vi "generate_random_rectangular_grid_and_word_list.vi"(7 "size (rows, columns)":i32[](array[numeric])=[300, 300], 9 "Min Word Length":u64=10, 10 "Max Word Length":u64=150, 11 "number of words":i32=300) -> (2 "Words":string[](array[string]), 3 "Grid":string[][](array[string]))   [LabVIEW 2020]
uses:
  <vilib>/numeric/Random Number (Range) U64.vi
  Letter Index--cluster.ctl
panel:
  # "From: Christian Altenbach\n https://forums.ni.com/t5/LabVIEW-Champions-Directory/LabVIEW-Champion-Christian-Altenbach/ta-p/3495223"
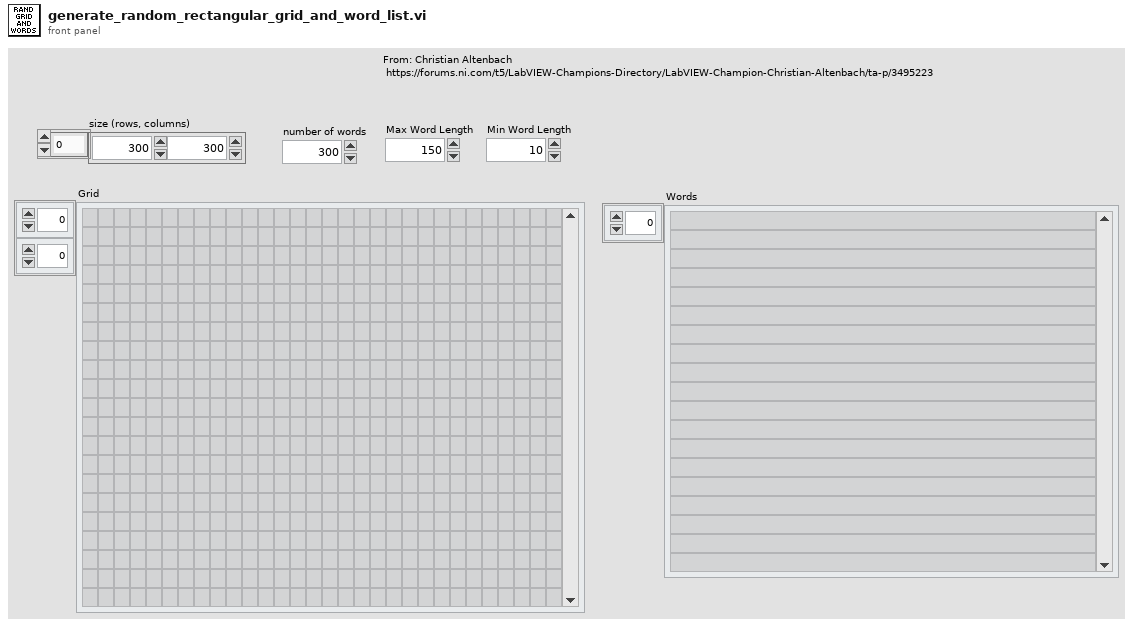
[diagram p1: front panel]
types:
  T1 = typedef "Letter Index--cluster.ctl" = cluster{"Row":i32, "Column":i32}
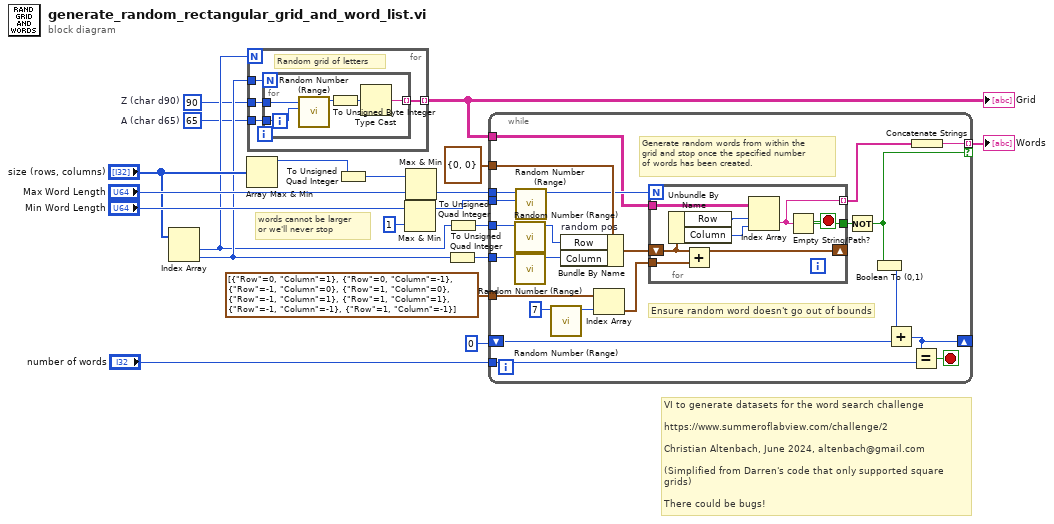
[diagram p0: block diagram]
diagram:
  w1 = u64 65  # A (char d65)
  w2 = u64 90  # Z (char d90)
  # "VI to generate datasets for the word search challenge\n\nhttps://www.summeroflabview.com/challenge/2\n\nChristian Altenbach, June 2024, altenbach@gmail.com\n\n(Simplified from Darren's code that only supported square grids)\n\nThere could be bugs!"
  # "words cannot be larger\nor we'll never stop"
  n1 = Index Array(array="size (rows, columns)") -> (element #1=w8:i32, element #2=w9:i32)  [unwired: 2 in]
  n2 = Array Max & Min(array="size (rows, columns)") -> (max value=w5:i32)  [unwired: 3 out]
  n3 = for {
    N: w8 -> [_]
    tunnel: [w24] -> w20 mode=indexing
    tunnel: w9 -> [w23]
    tunnel: w2 -> [w22]
    tunnel: w1 -> [w21]
    # "Random grid of letters"
    n4 = for {
      N: w23 -> [_]
      tunnel: [w27] -> w24 mode=indexing
      tunnel: w22 -> [w26]
      tunnel: w21 -> [w25]
      n5 = call-poly <vilib>:"Random Number (Range).vi"("lower bound (0)"=w25, "upper bound (100)"=w26) -> ("number"=w29:u64)  [unwired: 9 in]
      n6 = To Unsigned Byte Integer(number=w29) -> (unsigned 8bit integer=w28:u8)
      n7 = Type Cast(x=w28) -> (*(type *) &x=w27:string)  [unwired: 1 in]
    }
  }
  "Grid" <- w20
  n8 = To Unsigned Quad Integer(1:w5) -> (0:w15:u64)
  n9 = Max & Min(x="Min Word Length", y=u64 1) -> (max(x,y)=w7:u64)  [unwired: 1 out]
  n10 = Max & Min(x=w15, y="Max Word Length") -> (min(x,y)=w16:u64)  [unwired: 1 out]
  n11 = To Unsigned Quad Integer(1:w9) -> (0:w3:u64)
  n12 = To Unsigned Quad Integer(1:w8) -> (0:w4:u64)
  n13 = while {
    tunnel: w20 -> [w39]
    tunnel: "number of words" -> [w49]
    tunnel: w16 -> [w48]
    tunnel: w7 -> [w47]
    tunnel: T1 {"Row"=0, "Column"=0} ("Letter Index") -> [w45]
    tunnel: T1[] [{"Row"=0, "Column"=1}, {"Row"=0, "Column"=-1}, {"Row"=-1, "Column"=0}, {"Row"=1, "Column"=0}, {"Row"=-1, "Column"=1}, {"Row"=1, "Column"=1}, {"Row"=-1, "Column"=-1}, {"Row"=1, "Column"=-1}] -> [w44]
    tunnel: w4 -> [w42]
    tunnel: w3 -> [w41]
    shift-right: [w34] -> _
    shift-left: 0 -> [w35]
    tunnel: [w36] -> w10 mode=indexing if=w33
    stop <- w50 stop-if-true
    # "Ensure random word doesn't go out of bounds"
    # "Generate random words from within the\ngrid and stop once the specified number\nof words has been created."
    n14 = call-poly <vilib>:"Random Number (Range).vi"("upper bound (100)"=w42) -> ("number"=w52:u64)  [unwired: 10 in]
    n15 = call-poly <vilib>:"Random Number (Range).vi"("upper bound (100)"=w41) -> ("number"=w51:u64)  [unwired: 10 in]
    n16 = call-poly <vilib>:"Random Number (Range).vi"("lower bound (0)"=w47, "upper bound (100)"=w48) -> ("number"=w40:u64)  [unwired: 9 in]
    n17 = call-poly <vilib>:"Random Number (Range).vi"("upper bound (100)"=u64 7) -> ("number"=w46:u64)  [unwired: 10 in]
    n18 = Bundle By Name "random pos"(cluster=w45, "Row"=w52, "Column"=w51) -> (w43:T1)
    n19 = Index Array(array=w44, index=w46) -> (element=w38:T1)
    n20 = for {
      N: w40 -> [_]
      tunnel: w39 -> [w60]
      tunnel: w38 -> [w59]
      shift-right: [w58] -> _
      shift-left: w43 -> [w57]
      tunnel: [w54] -> w37 mode=indexing
      tunnel: [w53] -> w30
      stop <- w53 stop-if-true
      n21 = Unbundle By Name(w57) -> ("Row"=w56:i32, "Column"=w55:i32)
      n22 = Add(x=w57, y=w59) -> (x+y=w58:T1)
      n23 = Index Array(array=w60, index (row)=w56, index (col)=w55) -> (element=w54:string)
      n24 = Empty String/Path?(string/path=w54) -> (empty?=w53:bool)
    }
    n25 = Not(x=w30) -> (.not. x?=w33:bool)
    n26 = Boolean To (0,1)(Boolean=w33) -> (0, 1=w32:i16)
    n27 = Add(x=w32, y=w35) -> (x+y=w34:i32)
    n28 = Equal?(x=w34, y=w49) -> (x = y?=w50:bool)
    n29 = Concatenate Strings(w37) -> (w36:string)
  }
  "Words" <- w10
